vi "TachValue.vi"(9 "index":i32, 11 "array":string[](array[string])) -> (1 "Cluster":T1, 2 "Array":string[](array[string]), 3 "OUT First Value":string)   [LabVIEW 2017]
panel:
  out "element":u8
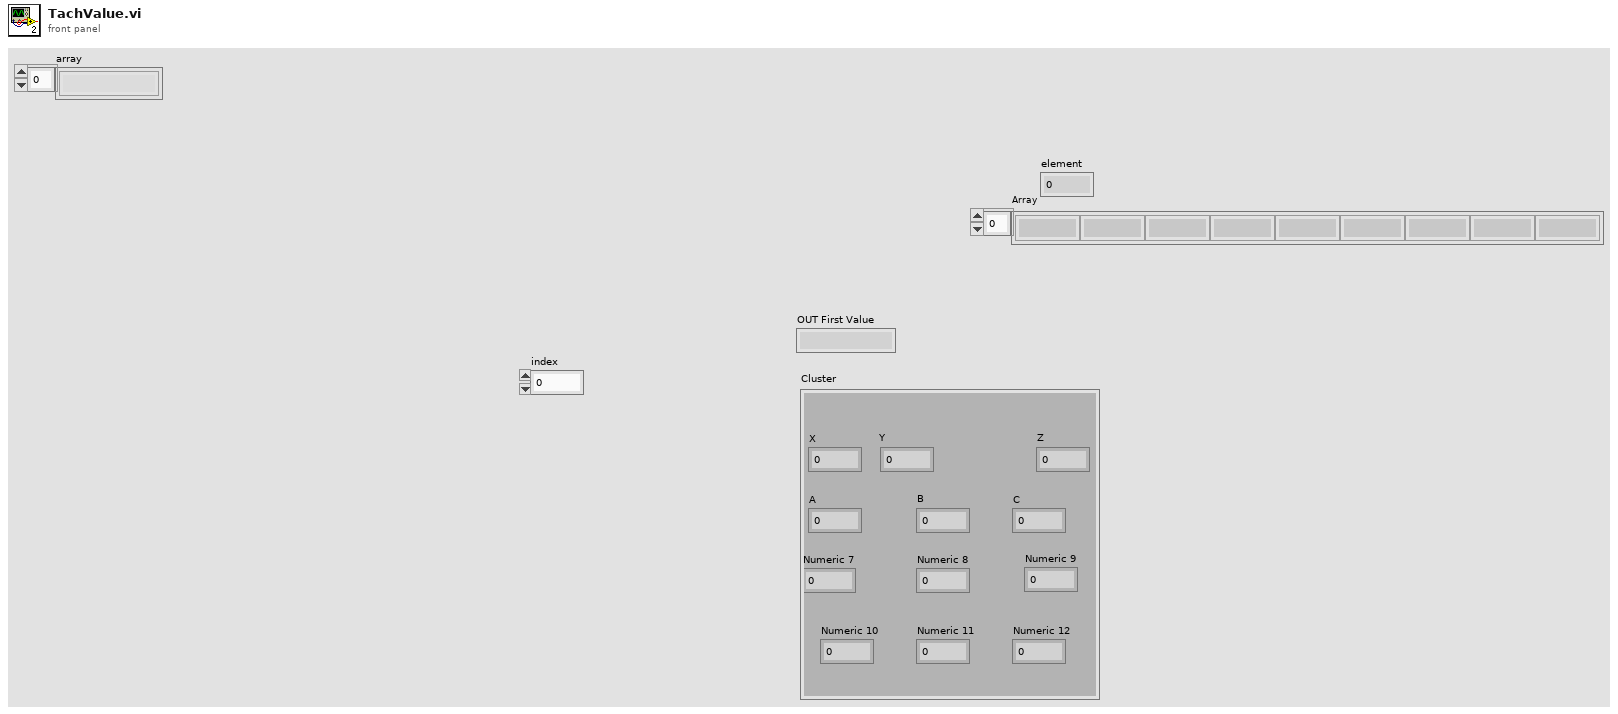
[diagram p1: front panel]
types:
  T1 = cluster{"X":dbl, "Y":dbl, "Z":dbl, "A":dbl, "B":dbl, "C":dbl, "Numeric 7":dbl, "Numeric 8":dbl, "Numeric 9":dbl, "Numeric 10":dbl, "Numeric 11":dbl, "Numeric 12":dbl}
  T2 = cluster{"array type (2D Dbl)[0]":dbl, "array type (2D Dbl)[1]":dbl, "array type (2D Dbl)[2]":dbl, "array type (2D Dbl)[3]":dbl, "array type (2D Dbl)[4]":dbl, "array type (2D Dbl)[5]":dbl, "array type (2D Dbl)[6]":dbl, "array type (2D Dbl)[7]":dbl, "array type (2D Dbl)[8]":dbl, "array type (2D Dbl)[9]":dbl, "array type (2D Dbl)[10]":dbl, "array type (2D Dbl)[11]":dbl}
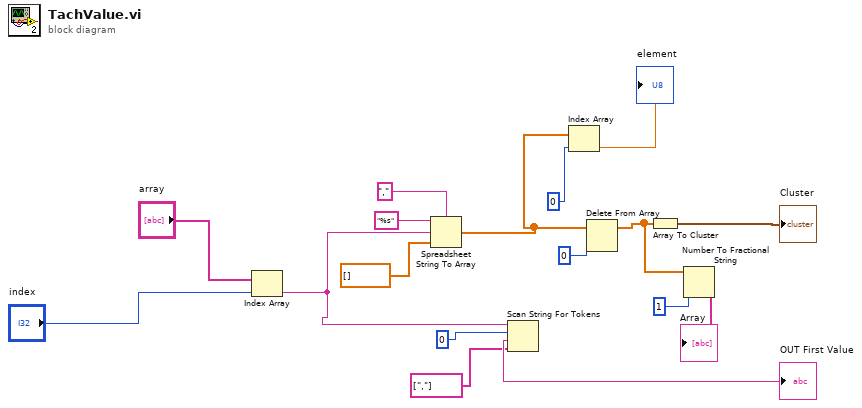
[diagram p0: block diagram]
diagram:
  n1 = Index Array(array="array", index="index") -> (element=w3:string)
  n2 = Spreadsheet String To Array(delimiter (Tab)=",", format string="%s", spreadsheet string=w3, array type (2D Dbl)=dbl[] []) -> (array=w4:dbl[])
  n3 = Scan String For Tokens(6:string[] [","] ("delimiters (\\s,\\t,\\r,\\n)"), 8:0 ("length (rest)"), 9:w3) -> (1:→"OUT First Value":string)  [unwired: 3 in, 3 out]
  n4 = Index Array "Index Array"(array=w4, index=0) -> (element=→"element":dbl)
  n5 = Delete From Array(array=w4, index=0) -> (array with subset deleted=w12:dbl[])  [unwired: 1 in, 1 out]
  n6 = Array To Cluster(array=w12) -> (cluster=→"Cluster":T2)
  n7 = Number To Fractional String(number=w12, precision (6)=i16 1) -> (F-format string=→"Array":string[])  [unwired: 2 in]
